vi "Tool data SIMULTERT gatheringloop.vi"(1 "Loop ID":T1, 11 "error out":errorcluster) -> ()   [LabVIEW 2011]
uses:
  Application Structure/Loop ID.ctl
  Modem Status/Variable List Modem Status Digital.ctl
  Tool/Variable List Tool Digital.ctl
  Common/Variable List Common Digital.ctl
  Modem Status/Variable List Modem Status Analog.ctl
  Tool/Variable List Tool Analog.ctl
  Common/Variable List Common Analog.ctl
  Action Analog Handler.ctl
  Status Digitalish.ctl
  emi Lib/System 01/0 - General/App/Loop control 2/Private/_emi_ SMLoop start condition.vi
  emi Lib/System 01/0 - General/App/Loop control 2/Private/_emi_ SMLoop Error Check.vi
  emi Lib/Basic/0 - General/Error/emi_Is Error.vi
  emi Lib/System 01/0 - General/App/Loop control 2/Private/_emi_SMLoop Register new.vi
  emi Lib/System 01/0 - General/S&E reporting/emi_Send S&E Error message.vi
  emi Lib/Basic/0 - General/Error/emi_ Is Error state.vi
  emi Lib/System 01/0 - General/emi_Read System ID.vi
  emi Lib/System 01/0 - General/App/Loop control/Private/_emi_GFV Loop Linking.vi
  emi Lib/System 01/0 - General/App/Loop control/Private/_emi_GFV Loop Enable.vi
  emi Lib/System 01/0 - General/App/Loop control 2/Private/_emi_ SMLoop Restart.vi
  emi Lib/System 01/0 - General/App/Private/_emi_GFV App Close.vi
  emi Lib/System 01/0 - General/App/Loop control 2/Private/_emi_ SMLoop Restart Counter.vi
  emi Lib/System 01/0 - General/App/Loop control/Private/_emi_GFV Loop Running.vi
  emi Lib/System 01/0 - General/Private/_emi_GFV System ID.vi
  emi Lib/System 01/0 - General/S&E reporting/Private/_emi_S&E Q Generator.vi
  <vilib>/Utility/error.llb/Clear Errors.vi
  emi Lib/System 01/0 - General/App/Loop control/Private/_emi_GFV stop a loop so it can reset.vi
  <vilib>/Utility/VariantDataType/GetNumericInfo.vi
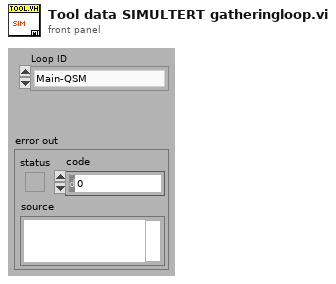
[diagram p1: front panel]
types:
  T1 = typedef "Loop ID.ctl" = enum16{"Main-QSM", "Main-Dialog", "Main-Ind Upd", "Main-Graph Upd", "Main-Debug", "Main-DebugW1", "Main-DebugW2", "Main-SE Handler", "Interface-PCP", "Interface-CANbus", "Interface-Modem", "Var Handling-Beat", "Var Handling-From PCP", "Var Handling-File storage", "Var Handling-From Simulator", "GUI-GrphW Mast", "GUI-GrphW Slav", "SIM-Tool W1", "SIM-Tool W2", "Alm-Sound", "LEIN-motor", "Tool data gatherer Qer", "Tool Data LEIN STAT2 dekoder", "Indicator Value Update", "Tool STAT2 dedicated reader", "Tool ID handler", "Detail View L1", "Detail View L2", "Main display enable view", "Sequence runner", "Voltage setpoint", "Resistance setpoint", "Stroker Wizard L1", "Stroker Wizard L2", "Alarm Handling", "Annotations Tip Strip", "Magna Interface", "Modem Status", "Var Handling - Modem Status", "Power interface detector"}
  T2 = typedef "Variable List Modem Status Digital.ctl" = enum16{"TMU_LINK_STATUS"}
  T3 = typedef "Variable List Tool Digital.ctl" = enum16{"Tool Error Controller", "Tool Stopped Controller", "Tool Relay 1", "Tool Relay 2", "Tool Both Relays", "Tool node Pressure 1", "Tool Error Pressure 1", "Tool Stopped Pressure 1", "Tool node Pressure 2", "Tool Error Pressure 2", "Tool Stopped Pressure 2", "Tool node Solenoid", "Tool Error Solenoid", "Tool Stopped Solenoid", "Tool Solenoid 1", "Tool Solenoid 2", "Tool Solenoid 3", "Tool node PSU", "Tool Error PSU", "Tool Stopped PSU", "Upper Tension Sub", "Tool Error Upper Tension Sub", "Tool Stopped Upper Tension Sub", "Lower Tension Sub", "Tool Error Lower Tension Sub", "Tool Stopped Lower Tension Sub", "Stroke Target seeking", "Stroke Moving Out", "Stroke Moving Inn", "Stroke valves set for Out", "Stroke valves set for In", "Stroke In (force)", "Stroke Out (force)", "Stroke Force decreasing(in)", "Stroke Force decreasing(out)", "Stroke Force change not correct", "Stroke SLIPS established P1", "Stroke SLIPS established P2", "Stroke SLIPS established", "Stroke Pressure Monitor Ongoing", "Stroke Pressure Monitor Ending ", "Tool Stroke enable Valve", "Tool Stroke direction Valve", "Tool Anchor Valve", "Stroker Var19 - Reserved", "Stroker Var20 - Reserved", "Stroker Var21 - Reserved", "Stroker Var22 - Reserved", "Stroker Var23 - Reserved", "Stroker Var24 - Reserved", "Tractor Var1 - Reserved", "Tractor Var2 - Reserved", "Tractor Var3 - Reserved", "Tractor Var4 - Reserved", "Tractor Var5 - Reserved", "Tractor Var6 - Reserved", "Tractor Var7 - Reserved", "Tractor Var8 - Reserved", "Oil filling mode", "Mill Bit Direction", "Position control", "Anchor", "Driller Var5 - Reserved", "Driller Var6 - Reserved", "Driller Var7 - Reserved", "Driller Var8 - Reserved"}
  T4 = typedef "Variable List Common Digital.ctl" = enum16{"PCP Connected", "PCP PC Control", "HV PSU connected", "HV PSU HV Active", "Modem Connected", "Tool Connected", "CanBus interface"}
  T5 = typedef "Variable List Modem Status Analog.ctl" = enum16{"TS_Signal_Quality", "TS_PCB_Temp", "TS_Gain", "DH_Signal_Quality", "DH_PCB_Temp", "DH_Gain", "Link_Status"}
  T6 = typedef "Variable List Tool Analog.ctl" = enum16{"Tool Max Temperature", "Tool (Controller) Temperature", "Tool Supply Voltage", "Tool (Controller) Current", "Tool Acceleration X", "Tool Acceleration Y", "Tool Acceleration Z", "Tool Acceleration Sum", "Tool Inclination", "Tool Rotation", "Tool GP Sensor 1", "Tool GP Sensor 2", "Tool (Pressure 1) Temperature", "Tool Pressure 1 RAW", "Tool (Pressure 2) Temperature", "Tool Pressure 2 RAW", "Tool (Solenoid) Temperature", "Tool Solenoid Position", "PSU Temp", "Head Voltage", "PSU Main Voltage out", "PSU Main Current out", "Upper Tension Sub Temp", "Tool Upper Tension Sub Raw", "Lower Tension Sub Temp", "Tool Lower Tension Sub Raw", "Tool Var27 - Reserved", "Tool Var28 - Reserved", "Tool Var29 - Reserved", "Tool Var30 - Reserved", "Stroke Extension", "Stroke In Force", "Stroke Out Force", "Stroke Force", "Stroker Pressure 1", "Stroker Pressure 2", "Stroker Upper Tension Sub", "Stroker Lower Tension Sub", "Stroker Var09 - Reserved", "Stroker Var10 - Reserved", "Tractor Upper Tension Sub", "Tractor Lower Tension Sub", "Tractor Var03 - Reserved", "Tractor Var04 - Reserved", "Tool Temperature sensor", "Tool Motor Voltage", "Tool Motor Current", "Tool Motor Torque", "Tool weight on bit", "Tool Motor RPM"}
  T7 = typedef "Variable List Common Analog.ctl" = enum16{"HVPSU Head Voltage", "HVPSU TS Voltage", "HVPSU Current", "PCP Cable Resistance", "Winch Depth", "Winch Line Speed", "Winch Wire Tension"}
  T8 = typedef "Action Analog Handler.ctl" = enum16{"GET value", "GET Single Frequenzy", "GET All Values", "GET Waveform", "Get Numb Var", "SET Value", "START Buffer", "REG Variable", "BUF size(total antal sekund)", "PULS", "Get a Value at time", "Set initial waveform"}
  T9 = typedef "Status Digitalish.ctl" = enum16{"NA", "False", "True"}
  T10 = typedef "_emi_ SMLoop sates.ctl" = enum16{"Init", "Standby", "Start", "Normal Operation", "Stop", "Error Handling", "End", "Post"}
  T11 = cluster{"Tool Data not":refnum<notifier>, "Tool Anal Size":i32, "Tool Dig Size":i32}
  T12 = typedef "Options  All pages and custom.ctl" = cluster{"P 1 (App)":T13, "P 2":T14, "P 3":T15, "P 4":T18, "P 5":T23, "P 6 (Err)":T24, "P 7 (Expert)":T25, "P 8 (Depth)":T27, "C 1":T28, "C 2":T29}
  T13 = typedef "Options Page 1 (App).ctl" = cluster{"Result files":path, "PCP Interface":string, "Tractor/Stroker Interface":string, "Tractor Interface":string, "Modem Status Interface":string, "Audible Alarm":bool, "Force alarm on Technical":bool, "Force alarm on HH":bool, "Force alarm on LL":bool, "Force alarm on H":bool, "Force alarm on L":bool}
  T14 = typedef "Options Page 2.ctl" = cluster{"Solenoid & Relay latching time":u16, "Tractor relay 1":dbl, "Tractor relay 2":dbl, "Tractor Solenoid limit":dbl}
  T15 = typedef "Options Page 3.ctl" = cluster{"Min resistance":dbl, "Max resistance":dbl, "Head voltage range":T16, "Max voltage jump":dbl, "Maximum resistance change":dbl, "Start Telemetry Voltage":dbl, "Start Telemetry Timeout":dbl, "Start Motor Voltage":dbl, "Stop Motor Voltage":dbl, "Pass Mode Warning Voltage":dbl, "Relay Switch Voltage":dbl, "Relay Status Loss Voltage":dbl, "Samples to average":i32, "PSU type DO NOT USE":T17, "Magna OVP":dbl, "Magna Current Limit":dbl}
  T16 = typedef "PCP type List.ctl" = enum16{"0 - 350V", "0 - 450V", "0 - 600V"}
  T17 = typedef "PSU Type.ctl" = enum16{"Unipower", "Magna 8.3A", "Magna 12A", "None"}
  T18 = typedef "Options Page 4.ctl" = cluster{"Solenoid & Relay latching time":u16, "Stroker relay 1":dbl, "Stroker Relay 2":dbl, "Stroker Solenoid limit":dbl, "Force det.":T19, "Stroke force lim.":dbl, "Anchor Enabled Pressure":dbl, "Tacometer puls":dbl, "Default anchor behavior":T20, "Default stroker behavior":T21, "Default stroker force limit (tonne)":dbl, "Slips Size":T22}
  T19 = typedef "Stroke force selector.ctl" = enum16{"Stroke in = node 1", "Strok out = node 1"}
  T20 = typedef "Default anchor behavior.ctl" = enum16{"Do nothing", "Set Anchor", "Release Anchor"}
  T21 = typedef "Default stroker behavior.ctl" = enum16{"Do nothing", "Stop", "Go Out", "Go In"}
  T22 = typedef "Slips Type Radio.ctl" = enum32{"No Selection", "338 MRS", "3,9 MRS"}
  T23 = typedef "Options Page 5.ctl" = cluster{"Solenoid & Relay latching time":u16, "Driller relay 1":dbl, "Driller Relay 2":dbl, "Driller  Solenoid limit":dbl}
  T24 = typedef "Options Page 6 (Err).ctl" = cluster{"Error and event files":path}
  T25 = typedef "Options Page 7 (Expert).ctl" = cluster{"Show Debug":bool, "Log debug messages":bool, "Additional debug messages":bool, "Start Beagle with Simulator data":bool, "Workshop mode":bool, "Modem baud":u16, "enumCANCOM":bool, "Modem sim":T26, "Telemetry Timeout Disable":i32, "Buffer size":i32, "Upd regular data":bool, "Cable comp":cluster{"VMOD1 Voltage(V)":dbl, "VMOD2 Voltage(V)":dbl}}
  T26 = typedef "Modem simulation setup.ctl" = cluster{"Modem dealay sim":bool, "Sim baud Tx":u16, "Bit Error fraction Tx":dbl, "Sim baud Rx":u16, "Bit Error fraction Rx":dbl}
  T27 = typedef "Options Page 8 (Depth).ctl" = cluster{"Winch Spool Circumference":dbl, "Winch Pulses per Revolution":dbl, "Current Depth":dbl}
  T28 = typedef "Options Custom 1.ctl" = cluster{"Depth Updated":bool, "Depth Offset":dbl}
  T29 = typedef "Options Custom 2.ctl" = cluster{"Placeholder":bool}
  T30 = typedef "Fixed Analog Channel Definition.ctl" = cluster{"ID":u16, "Name":string, "Quantity":T31, "Unit":string, "Maximum upd":T32, "Comment":string, "Help file Name":string, "Help file Section ":string, "Category":T33, "User adjustable Scaling":bool, "Default Scaling":T34, "Default Unit":i32, "Classification":T35}
  T31 = typedef "Quantity enum.ctl" = enum16{"NA", "Acceleration", "Angle", "Current", "Force", "Distance", "Pressure", "Resistance", "Rotational Speed", "Speed", "Temperature", "Tension", "Torque", "Voltage", "Weight"}
  T32 = typedef "Update frequensies.ctl" = enum16{"2 Hz", "1 Hz", "0.1 Hz"}
  T33 = typedef "Channel catagory Enum.ctl" = enum16{"No Category", "Power", "Temperature", "Pressure"}
  T34 = typedef "Scaling.ctl" = cluster{"Gain":dbl, "Offset":dbl}
  T35 = typedef "Channel Classification Enum.ctl" = enum16{"Basic", "Advanced", "Expert", "Unused"}
  T36 = typedef "Fixed Digital Channel Definition.ctl" = cluster{"ID":u16, "Name":string, "NA Text":string, "Off Text":string, "On Text":string, "Maximum upd":T32, "Comment":string, "Help file Name":string, "Help file Section ":string, "Catagory":T33, "In use":bool}
  T37 = typedef "Tool simulator data.ctl" = cluster{"Analog Values":dbl[], "Digital Values":T9[]}
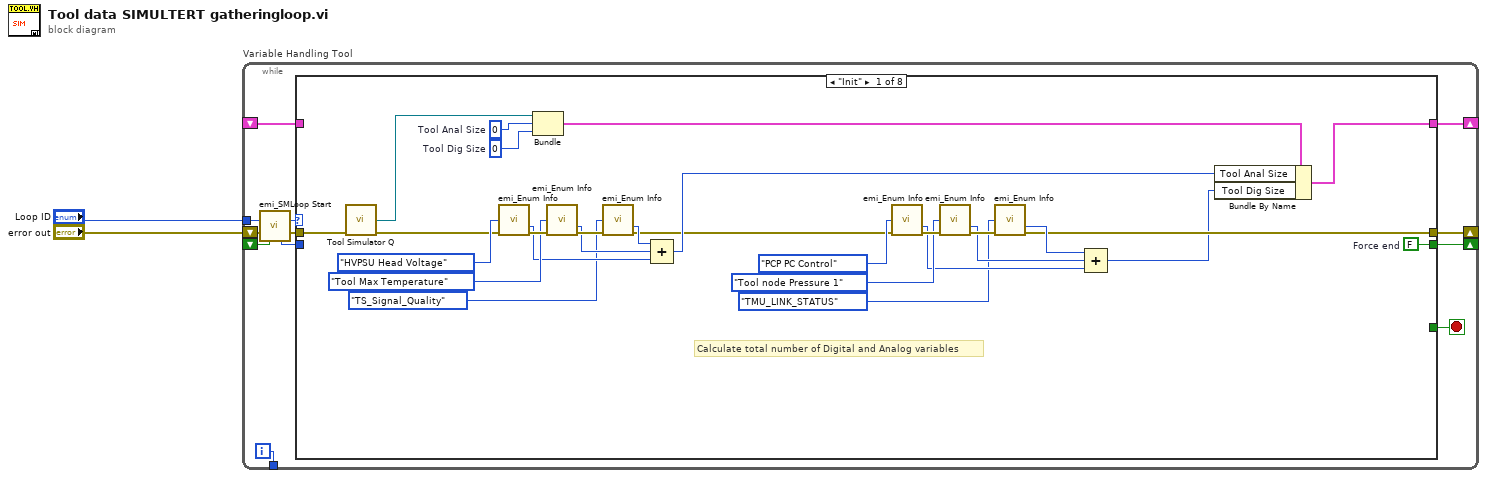
[diagram p0: block diagram]
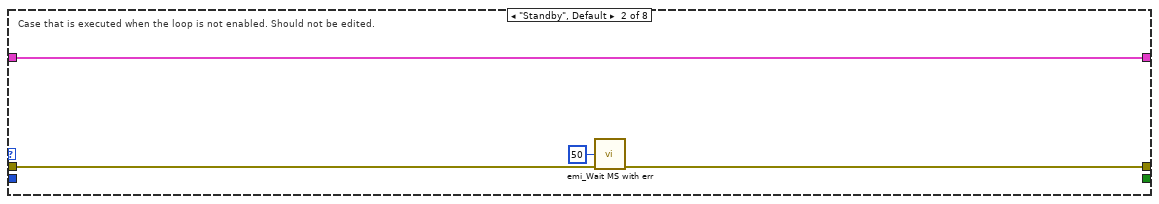
[diagram p2: hidden frame]
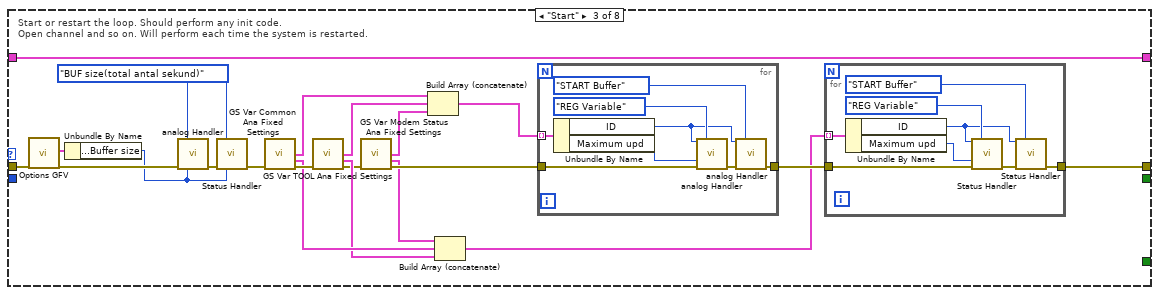
[diagram p3: hidden frame]
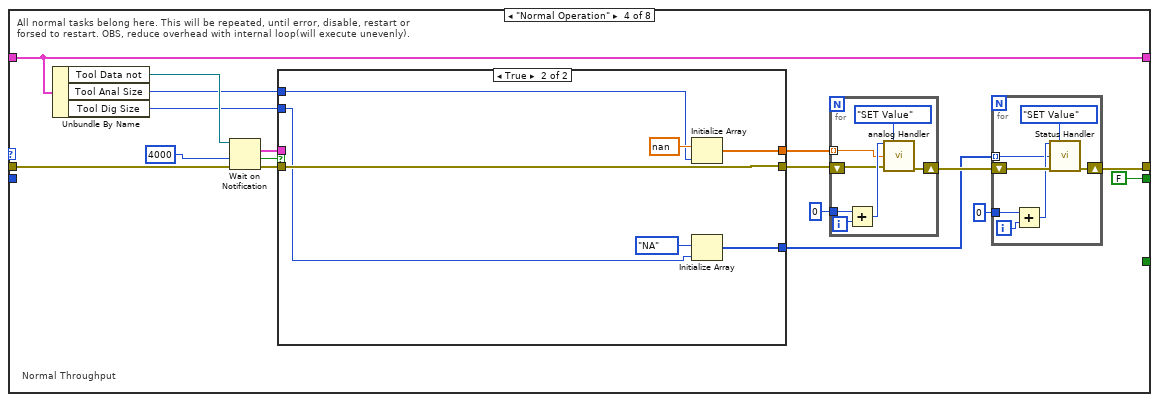
[diagram p4: hidden frame]
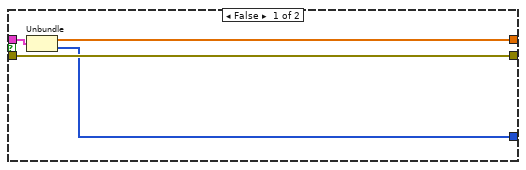
[diagram p5: hidden frame]
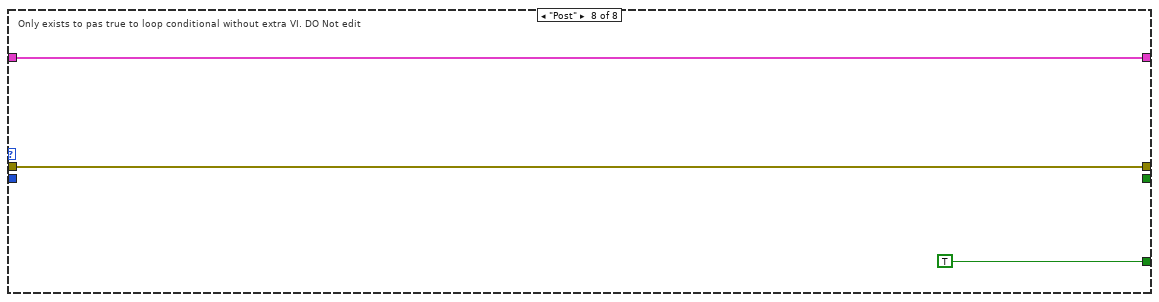
[diagram p9: hidden frame]
diagram:
  n1 = while "Variable Handling Tool" {
    shift-right: [w14] -> _
    shift-left: _ -> [w10]
    shift-right: [w12] -> _
    shift-left: "error out" -> [w8]
    tunnel: [w11] -> _
    shift-right: [w9] -> _
    shift-left: _ -> [w4]
    tunnel: "Loop ID" -> [w5]
    i -> [w11]
    stop <- w13 stop-if-true
    n2 = call "emi_SMLoop Start.vi"("Loop ID"=w5, "error in (no error)"=w8, "Force Stop(F)"=w4) -> ("Loop command"=w6:T10, "error out"=w7:errorcluster, "Loop ID out"=w3:i32)  [unwired: 10 in]
    n3 = case shown="\"Init\"" w6 {
      tunnel: [w38 w43 w64 w99 w126 w129 w130 w133] -> w14
      tunnel: [_ _ _ _ _ _ _ TRUE] -> w13
      tunnel: w7 -> [w40 w45 w65 w86 w127 w128 w131 w134]
      tunnel: [w16 w44 w59 w100 w127 w128 w131 w134] -> w12
      tunnel: w10 -> [_ w43 w64 w99 w126 w129 w130 w133]
      tunnel: [w41 _ _ FALSE ("Force End") _ _ _ _] -> w9
      tunnel: w3 -> [_ _ _ _ _ _ _ _]
      frame "Init" {
        w36 = 0  # Tool Dig Size
        w37 = 0  # Tool Anal Size
        w41 = FALSE  # Force end
        # "Calculate total number of Digital and Analog variables"
        n4 = call "Tool Simulator Q.vi"("error in (no error)"=w40) -> ("Tool Data not"=w39:refnum<notifier>, "error out"=w27:errorcluster)  [unwired: 12 in, 1 out]
        n5 = call "emi_Enum Info.vi"("Enum"=Variable_List_Common_Analog."HVPSU Head Voltage" ("First part list"), "error in (no error)"=w27) -> ("Numb Elements"=w29:i32, "error out"=w35:errorcluster)  [unwired: 10 in, 2 out]
        n6 = Bundle("Tool Data not"=w39, "Tool Anal Size"=w37, "Tool Dig Size"=w36) -> (w42:T11)  [unwired: 1 in]
        n7 = call "emi_Enum Info.vi"("Enum"=Variable_List_Tool_Analog."Tool Max Temperature" ("Variable ID"), "error in (no error)"=w35) -> ("Numb Elements"=w30:i32, "error out"=w32:errorcluster)  [unwired: 10 in, 2 out]
        n8 = call "emi_Enum Info.vi"("Enum"=Variable_List_Modem_Status_Analog."TS_Signal_Quality" ("Variable ID"), "error in (no error)"=w32) -> ("Numb Elements"=w31:i32, "error out"=w17:errorcluster)  [unwired: 10 in, 2 out]
        n9 = Compound Arithmetic op=ADD(w31, w30, w29) -> (w26:i32)
        n10 = call "emi_Enum Info.vi"("Enum"=Variable_List_Common_Digital."PCP PC Control" ("Action"), "error in (no error)"=w17) -> ("Numb Elements"=w19:i32, "error out"=w25:errorcluster)  [unwired: 10 in, 2 out]
        n11 = call "emi_Enum Info.vi"("Enum"=Variable_List_Tool_Digital."Tool node Pressure 1", "error in (no error)"=w25) -> ("Numb Elements"=w20:i32, "error out"=w22:errorcluster)  [unwired: 10 in, 2 out]
        n12 = call "emi_Enum Info.vi"("Enum"=Variable_List_Modem_Status_Digital."TMU_LINK_STATUS", "error in (no error)"=w22) -> ("Numb Elements"=w21:i32, "error out"=w16:errorcluster)  [unwired: 10 in, 2 out]
        n13 = Compound Arithmetic op=ADD(w21, w20, w19) -> (w15:i32)
        n14 = Bundle By Name(cluster=w42, "Tool Anal Size"=w26, "Tool Dig Size"=w15) -> (w38:T11)
      }
      frame "Standby", Default {
        # "Case that is executed when the loop is not enabled. Should not be edited."
        n15 = call "emi_Wait MS with err.vi"("milliseconds to wait(0)"=u32 50, "error in (no error)"=w45) -> ("error out"=w44:errorcluster)  [unwired: 13 in]
      }
      frame "Start" {
        w62 = Action_Analog_Handler."BUF size(total antal sekund)" ("Action(GET)")
        # "Start or restart the loop. Should perform any init code. \nOpen channel and so on. Will perform each time the system is restarted."
        n16 = call "Options GFV.vi"("error in (no error)"=w65) -> ("Options"=w66:T12, "error out"=w67:errorcluster)  [unwired: 16 in, 1 out]
        n17 = Unbundle By Name(w66) -> ("P 7 (Expert).Buffer size"=w61:i32)
        n18 = call "analog Handler.vi"("Action"=w62, "error in (no error)"=w67, "Start tid / buf size"=w61) -> ("error out"=w63:errorcluster)  [unwired: 7 in, 5 out]
        n19 = call "Status Handler.vi"("Action"=w62, "error in (no error)"=w63, "Start tid(buff size"=w61) -> ("error out"=w58:errorcluster)  [unwired: 8 in, 4 out]
        n20 = call "GS Var Common Ana Fixed Settings.vi"("error in (no error)"=w58) -> ("Common Analog Var Fixed out"=w56:T30[], "Common Digital var Fixed"=w53:T36[], "error out"=w57:errorcluster)  [unwired: 12 in]
        n21 = call "GS Var TOOL Ana Fixed Settings.vi"("error in (no error)"=w57) -> ("Tool Analog var Fixed out"=w55:T30[], "Tool Digital Var Fixed out"=w52:T36[], "error out"=w50:errorcluster)  [unwired: 12 in]
        n22 = call "GS Var Modem Status Ana Fixed Settings.vi"("error in (no error)"=w50) -> ("Modem Status Analog var Fixed out"=w48:T30[], "Modem Status Digital Var Fixed out"=w47:T36[], "error out"=w49:errorcluster)  [unwired: 12 in]
        n23 = Build Array (concatenate)(w56, w55, w48) -> (w54:T30[])
        n24 = Build Array (concatenate)(w47, w53, w52) -> (w51:T36[])
        n25 = for {
          tunnel: [w78] -> w60
          tunnel: w49 -> [w83]
          tunnel: w54 -> [w82] mode=indexing
          n26 = Unbundle By Name(w82) -> ("ID"=w76:u16, "Maximum upd"=w81:T32)
          n27 = call "analog Handler.vi"("Variable Index"=w76, "Action"=Action_Analog_Handler."REG Variable" ("Action(GET)"), "Upd freq"=w81, "error in (no error)"=w83) -> ("error out"=w79:errorcluster)  [unwired: 6 in, 5 out]
          n28 = call "analog Handler.vi"("Variable Index"=w76, "Action"=Action_Analog_Handler."START Buffer" ("Action(GET)"), "error in (no error)"=w79) -> ("error out"=w78:errorcluster)  [unwired: 7 in, 5 out]
        }
        n29 = for {
          tunnel: [w70] -> w59
          tunnel: w60 -> [w75]
          tunnel: w51 -> [w74] mode=indexing
          n30 = Unbundle By Name(w74) -> ("ID"=w68:u16, "Maximum upd"=w73:T32)
          n31 = call "Status Handler.vi"("Variable Index"=w68, "Action"=Action_Analog_Handler."REG Variable" ("Action(GET)"), "Upd freq"=w73, "error in (no error)"=w75) -> ("error out"=w71:errorcluster)  [unwired: 7 in, 4 out]
          n32 = call "Status Handler.vi"("Variable Index"=w68, "Action"=Action_Analog_Handler."START Buffer" ("Action(GET)"), "error in (no error)"=w71) -> ("error out"=w70:errorcluster)  [unwired: 8 in, 4 out]
        }
      }
      frame "Normal Operation" {
        # "Normal Throughput"
        # "All normal tasks belong here. This will be repeated, until error, disable, restart or\nforsed to restart. OBS, reduce overhead with internal loop(will execute unevenly)."
        n33 = Unbundle By Name(w99) -> ("Tool Data not"=w97:refnum<notifier>, "Tool Anal Size"=w85:i32, "Tool Dig Size"=w84:i32)
        n34 = Wait on Notification(notifier=w97, timeout in ms (-1)=4000 ("P 7 (Expert).Telemetry Timeout Disable"), error in (no error)=w86) -> (notification=w94:T37, timed out?=w95:bool, error out=w96:errorcluster)  [unwired: 1 in, 1 out]
        n35 = case shown="True" w95 {
          tunnel: w96 -> [w116 w121]
          tunnel: w94 -> [w118 _]
          tunnel: [w117 w124] -> w93
          tunnel: [w116 w121] -> w92
          tunnel: [w115 w122] -> w88
          tunnel: w85 -> [_ w120]
          tunnel: w84 -> [_ w119]
          frame False {
            n36 = Unbundle(w118) -> ("Analog Values"=w117:dbl[], "Digital Values"=w115:T9[])
          }
          frame True {
            n37 = Initialize Array(nan ("element"), w120) -> (w124:dbl[])
            n38 = Initialize Array(Status_Digitalish."NA" ("Status in"), w119) -> (w122:T9[])
          }
        }
        n39 = for {
          tunnel: w93 -> [w111] mode=indexing
          tunnel: 0 ("Ana com") -> [w108]
          shift-right: [w109] -> w91
          shift-left: w92 -> [w110]
          i -> [w114]
          n40 = Add(x=w108, y=w114) -> (x+y=w112:i32)
          n41 = call "analog Handler.vi"("Variable Index"=w112, "Action"=Action_Analog_Handler."SET Value" ("Action(GET)"), "Value"=w111, "error in (no error)"=w110) -> ("error out"=w109:errorcluster)  [unwired: 6 in, 5 out]
        }
        n42 = for {
          shift-right: [w107] -> w100
          shift-left: w91 -> [w106]
          tunnel: 0 ("Ana com") -> [w103]
          tunnel: w88 -> [w101] mode=indexing
          i -> [w104]
          n43 = Add(x=w103, y=w104) -> (x+y=w102:i32)
          n44 = call "Status Handler.vi"("Variable Index"=w102, "Action"=Action_Analog_Handler."SET Value", "Value"=w101, "error in (no error)"=w106) -> ("error out"=w107:errorcluster)  [unwired: 7 in, 4 out]
        }
      }
      frame "Stop" {
        # "Stop the loop. May be restarted later. Close interfaces and the like"
      }
      frame "Error Handling" {
        # "Loop automaticaly returns here after error is found. If error is cleared, \nLoop wil continue as normal(if was operative when error."
      }
      frame "End" {
        # "Only executes at application end has. Should performa any action the loop \nneeds to finnish. Executes only once."
      }
      frame "Post" {
        # "Only exists to pas true to loop conditional without extra VI. DO Not edit"
      }
    }
  }
